vi "Voltage Pulse Gating System (HV supply).vi"(8 "error in (no error)":errorcluster, 10 "Pulse Gating System (HV supply).lvclass":refnum<class "Pulse Gating System (HV supply).lvclass">, 11 "Voltage Pulse Gating System (HV supply) in":refnum<class "Voltage Pulse Gating System (HV supply).lvclass">) -> (0 "error out":errorcluster, 3 "Voltage Pulse Gating System (HV supply) out":refnum<class "Voltage Pulse Gating System (HV supply).lvclass">)   [LabVIEW 2017, in "Voltage Pulse Gating System (HV supply).lvclass"]
uses:
  Voltage Pulse Gating System (HV supply).lvclass
  C:/LabVIEW-programs/Scanners/Scanner/Scanner.lvclass
  Instruments/Pusle Gating System (HV supply)/Pulse Gating System (HV supply).lvclass
  C:/LabVIEW-programs/Instruments/Utility Classes/Scannable/Scannable.lvclass
  Scanner/Scanner.lvclass
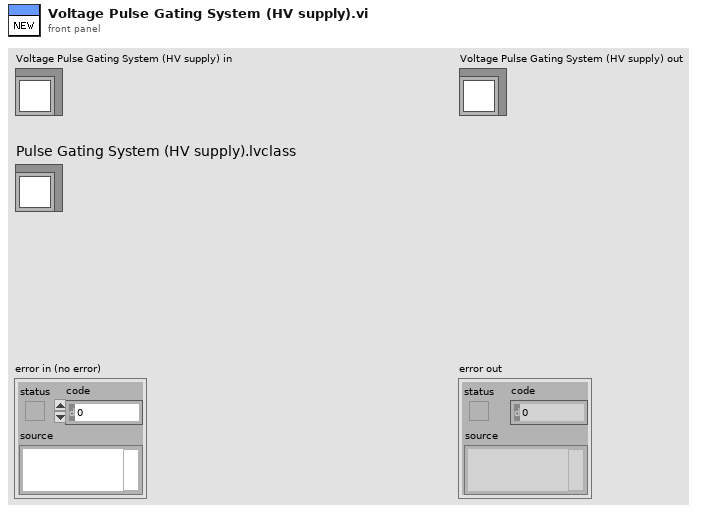
[diagram p1: front panel]
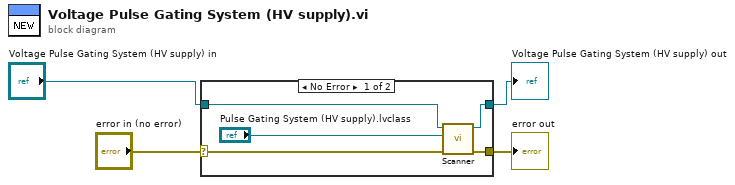
[diagram p0: block diagram]
diagram:
  n1 = case shown="No Error" "error in (no error)" {
    selector: "error in (no error)" -> [w9 w11]
    tunnel: [w6 w11] -> w2
    tunnel: [w8 w10] -> w1
    tunnel: "Voltage Pulse Gating System (HV supply) in" -> [w7 w10]
    frame No Error {
      n2 = call "Scanner.vi"("error in (no error)"=w9, "Scannable"="Pulse Gating System (HV supply).lvclass", "Scanner.lvclass in"=w7) -> ("error out"=w6:errorcluster, "Scanner.lvclass out"=w8:refnum<class "Voltage Pulse Gating System (HV supply).lvclass">)  [unwired: 1 in, 6 out]
    }
    frame Error {
    }
  }
  "error out" <- w2
  "Voltage Pulse Gating System (HV supply) out" <- w1
